vi "3.保存Log到文件.vi"(8 "error in":errorcluster, 11 "Module ID":i32=-1) -> (0 "error out":errorcluster)   [LabVIEW 2020, in "Log.lvlib"]
uses:
  Log.lvlib
  Log.lvlibp
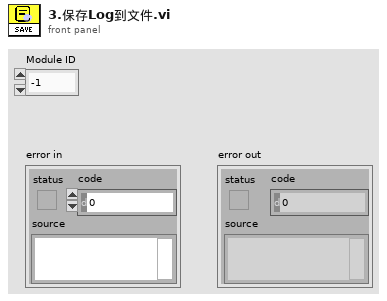
[diagram p1: front panel]
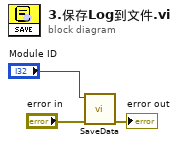
[diagram p0: block diagram]
diagram:
  n1 = call "SaveData.vi"("error in"="error in", "Module ID"="Module ID") -> ("error out"=→"error out":errorcluster)  [unwired: 9 in]
